vi "Example Bundler 1.vi"() -> ()   [LabVIEW 2014]
panel:
  out "ClusterIndicatorMy":cluster{string, i32, string[]}
  out "Error Out":errorcluster
  in  "Error In":errorcluster
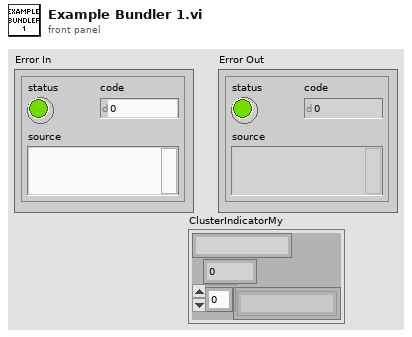
[diagram p1: front panel]
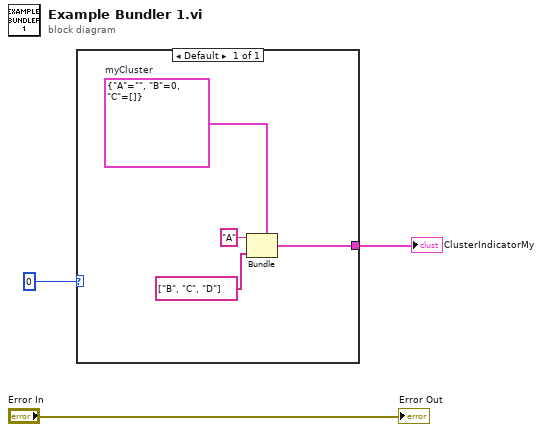
[diagram p0: block diagram]
diagram:
  n1 = case shown="Default" 0 {
    tunnel: [w5] -> w1
    frame Default {
      w4 = cluster{"A":string, "B":i32, "C":string[]} {"A"="", "B"=0, "C"=[]}  # myCluster
      n2 = Bundle(cluster=w4, "A"="A", "C"=string[] ["B", "C", "D"]) -> (w5:cluster{"A":string, "B":i32, "C":string[]})  [unwired: 1 in]
    }
  }
  "ClusterIndicatorMy" <- w1
  "Error Out" <- "Error In"
